vi "Set Goal A.vi"(11 "GIC Input":T1={"     Use ?\nOff       On"=[FALSE, TRUE, FALSE, TRUE], "Mode:"=FALSE, "Extra Port"="", "Hokuyo Port"="COM7", "Tx Prop  Port"="COM6", "Compass Port"="", "GPS Port"="", "Num of WPs"=0, "WP Lats and Longs"={"WP Lats"=[], "WP Longs"=[]}, "Obst Lats and Longs"={"Obst Lats"=[], "Obst Longs"=[]}, "Parameters"=[], "GPS Data"=[], "Compass"=0.0, "LMS Vector"=[], "Vision Vector"=[], "Direction Cmd"=0.0, "Speed Cmd"=0.0, "WP Vector"=[], "WP Number"=0, "Extra"=0, "SW Map"=[], "Path Cluster"={"Path x node"=[], "Path y node"=[]}, "Sim Course"=[]} {"Obst Lats and Longs"."Obst Longs" format="%#_8g"; "Obst Lats and Longs"."Obst Lats" format="%#_8g"}) -> (3 "GIC Output":T1={"     Use ?\nOff       On"=[FALSE, TRUE, FALSE, TRUE], "Mode:"=FALSE, "Extra Port"="", "Hokuyo Port"="COM7", "Tx Prop  Port"="COM6", "Compass Port"="", "GPS Port"="", "Num of WPs"=0, "WP Lats and Longs"={"WP Lats"=[], "WP Longs"=[]}, "Obst Lats and Longs"={"Obst Lats"=[], "Obst Longs"=[]}, "Parameters"=[], "GPS Data"=[], "Compass"=0.0, "LMS Vector"=[], "Vision Vector"=[], "Direction Cmd"=0.0, "Speed Cmd"=0.0, "WP Vector"=[], "WP Number"=0, "Extra"=0, "SW Map"=[], "Path Cluster"={"Path x node"=[], "Path y node"=[]}, "Sim Course"=[]} {"Obst Lats and Longs"."Obst Longs" format="%#_8g"; "Obst Lats and Longs"."Obst Lats" format="%#_8g"})   [LabVIEW 2014]
panel:
  out "tp":dbl
  out "wp vector":dbl[](array[numeric])
  out "test":dbl
  out "goal y":dbl
  in  "WP Vector":dbl[](array[numeric])=[-30.0, 100.0]
  out "goal x":dbl
  out "Test Output SWMap":dbl[][](array[numeric])
  in  "WayPoint:":dbl=100.0
  in  "Distance:":dbl=50.0
  in  "Slant:":dbl
  in  "Gap:":dbl=50.0
  in  "Ahead:":dbl
  # "Set Goal A"
  # "Input:"
  # "Output:"
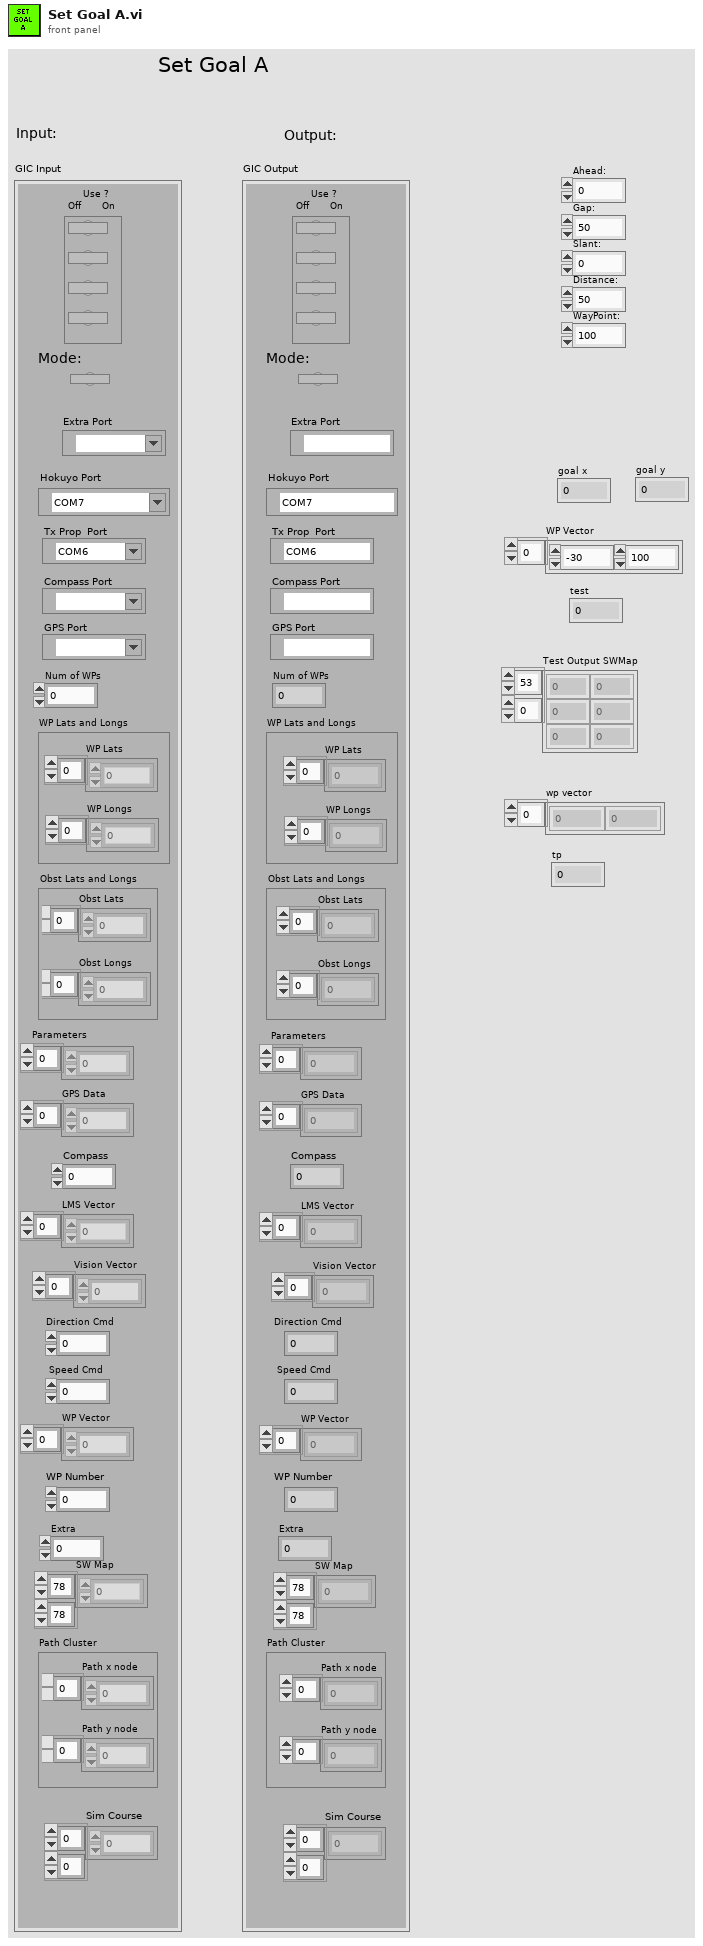
[diagram p1: front panel]
types:
  T1 = cluster{"     Use ?\nOff       On":bool[], "Mode:":bool, "Extra Port":refnum<visa-resource-name>, "Hokuyo Port":refnum<visa-resource-name>, "Tx Prop  Port":refnum<visa-resource-name>, "Compass Port":refnum<visa-resource-name>, "GPS Port":refnum<visa-resource-name>, "Num of WPs":i16, "WP Lats and Longs":cluster{"WP Lats":dbl[], "WP Longs":dbl[]}, "Obst Lats and Longs":cluster{"Obst Lats":dbl[], "Obst Longs":dbl[]}, "Parameters":dbl[], "GPS Data":dbl[], "Compass":dbl, "LMS Vector":dbl[], "Vision Vector":dbl[], "Direction Cmd":dbl, "Speed Cmd":dbl, "WP Vector":dbl[], "WP Number":i32, "Extra":i16, "SW Map":i32[][], "Path Cluster":cluster{"Path x node":dbl[], "Path y node":dbl[]}, "Sim Course":i8[][]}
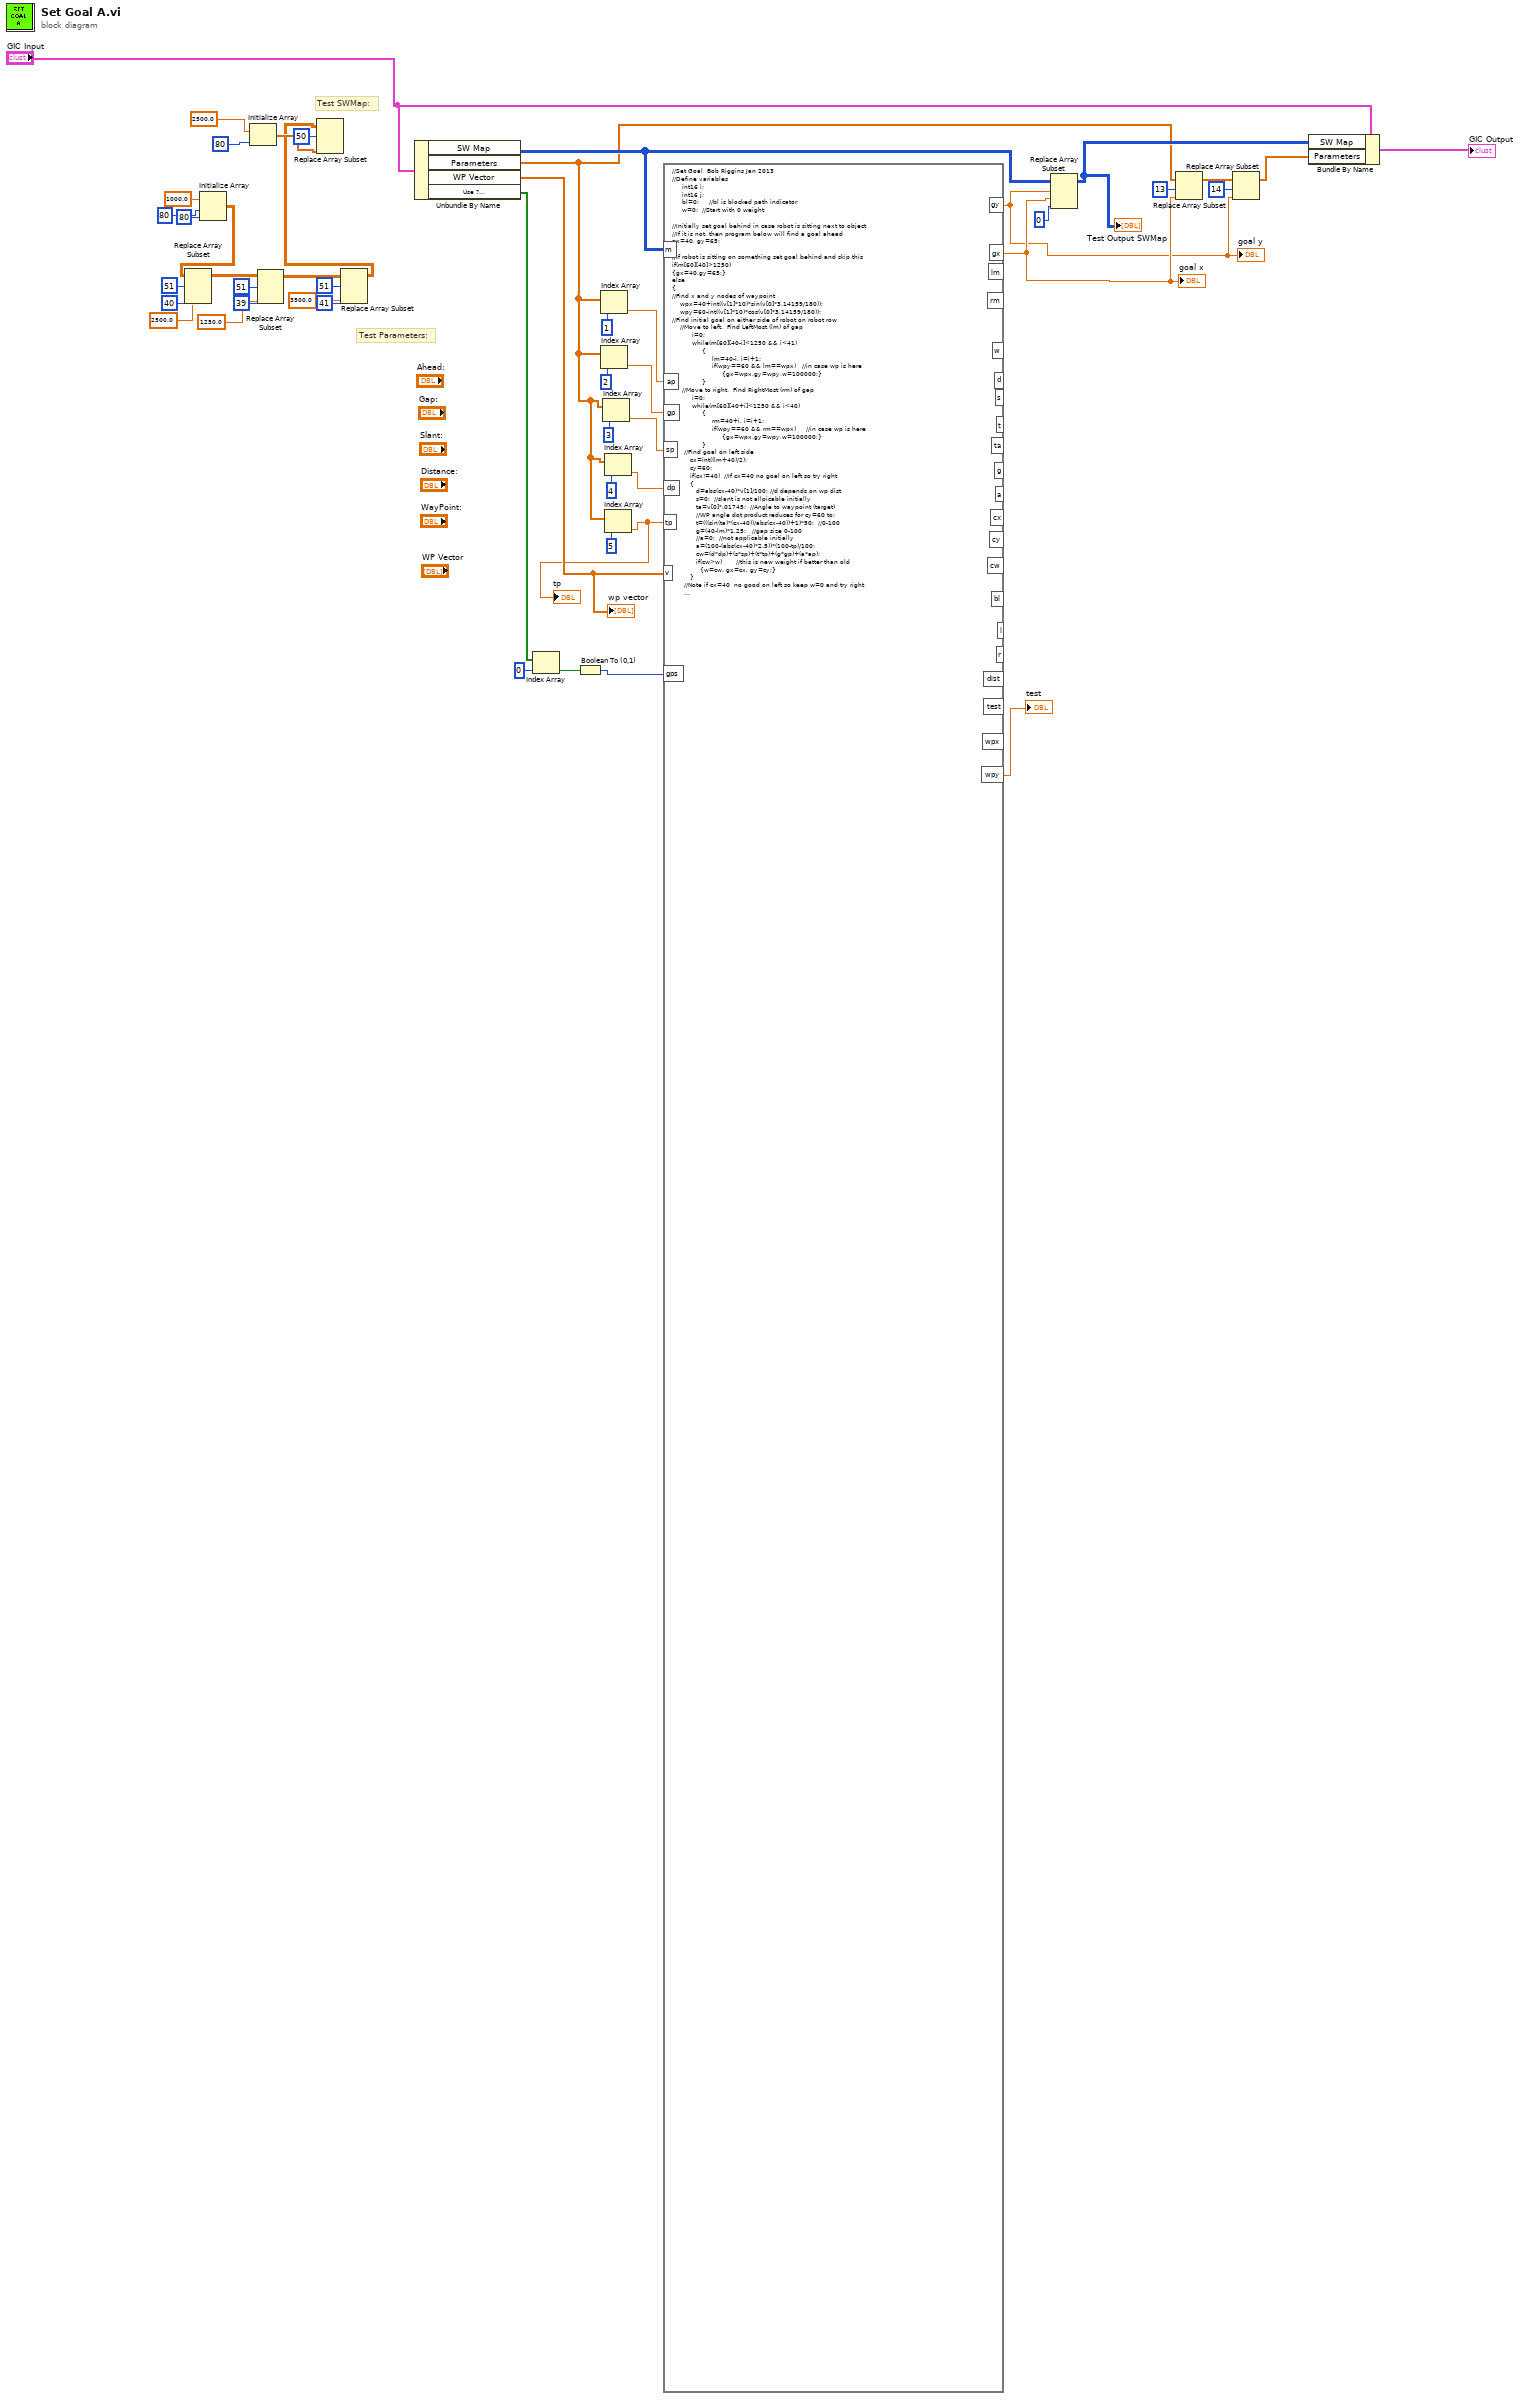
[diagram p0: block diagram]
diagram:
  # "Test Parameters:"
  # "Test SWMap:"
  n1 = Initialize Array(1000.0 ("element"), 80 ("dimension size"), 80 ("dimension size")) -> (w29:dbl[][])
  n2 = Replace Array Subset(array=w29, new element=2500.0 ("new element/subarray"), index (row)=51, index (col)=40 ("disabled index (col)")) -> (w42:dbl[][])
  n3 = Initialize Array(2500.0 ("element"), 80 ("dimension size")) -> (w31:dbl[])
  n4 = Replace Array Subset(array=w42, new element=1250.0 ("new element/subarray"), index (row)=51, index (col)=39 ("disabled index (col)")) -> (w38:dbl[][])
  n5 = Replace Array Subset(array=w38, new element=3500.0 ("new element/subarray"), index (row)=51, index (col)=41 ("disabled index (col)")) -> (w28:dbl[][])
  n6 = Replace Array Subset(array=w28, new element=w31, index (row)=50) -> ()  [unwired: 1 in, 1 out]
  n7 = Unbundle By Name("GIC Input") -> ("SW Map"=w25:i32[][], "Parameters"=w15:dbl[], "WP Vector"=w8:dbl[], "Use ?\nOff       On"=w6:bool[])
  "wp vector" <- w8
  n8 = Index Array(array=w6, index=0) -> (element=w4:bool)
  n9 = Boolean To (0,1)(Boolean=w4) -> (0, 1=w3:i16)
  n10 = Index Array(array=w15, index=1) -> (element=w24:dbl)
  n11 = Index Array(array=w15, index=2) -> (element=w21:dbl)
  n12 = Index Array(array=w15, index=3) -> (element=w19:dbl)
  n13 = Index Array(array=w15, index=4) -> (element=w17:dbl)
  n14 = Index Array(array=w15, index=5) -> (element=w7:dbl)
  "tp" <- w7
  n15 = formula code="//Set Goal  Bob Riggins Jan 2013\n//Define variables\n     int16 i;\n     int16 j;\n     bl=0;     //bl is blocked path indicator\n     w=0;  //Start with 0 weight\n\n//Initially set goal behind in case robot is sitting next to object\n//If it is not, then program below will find a goal ahead\ngx=40, gy=65;\n\n//If robot is sitting on something set goal behind and skip this\nif(m[60][40]>1250)\n{gx=40,gy=65;}\nelse\n{\n//Find x and y nodes of waypoint\n    wpx=40+int((v[1]*10)*sin(v[0]*3.14159/180));\n    wpy=60-int((v[1]*10)*cos(v[0]*3.14159/180));\n//Find initial goal on either side of robot on robot row\n    //Move to left.  Find LeftMost (lm) of gap\n          i=0;\n          while(m[60][40-i]<1250 && i<41)\n               {\n                    lm=40-i, i=i+1;\n                    if(wpy==60 && lm==wpx)   //in case wp is here\n                         {gx=wpx,gy=wpy,w=100000;}\n               }\n     //Move to right.  Find RightMost (rm) of gap\n          i=0;\n          while(m[60][40+i]<1250 && i<40)\n               {\n                    rm=40+i, i=i+1;\n                    if(wpy==60 && rm==wpx)     //in case wp is here\n                         {gx=wpx,gy=wpy,w=100000;}\n               }\n      //Find goal on left side\n         cx=int((lm+40)/2);\n         cy=60;\n         if(cx!=40)  //If cx=40 no goal on left so try right\n         {\n            d=abs(cx-40)*v[1]/100; //d depends on wp dist\n            s=0;  //slant is not allpicable initially\n            ta=v[0]*.01745;  //Angle to waypoint (target)\n            //WP angle dot product reduces for cy=60 to:\n            t=(((sin(ta)*(cx-40))/abs(cx-40))+1)*50;  //0-100\n            g=(40-lm)*1.25;   //gap size 0-100\n            //a=0;  //not applicable initially\n            a=(100-(abs(cx-40)*2.5))*(100-tp)/100;\n            cw=(d*dp)+(s*sp)+(t*tp)+(g*gp)+(a*ap);\n            if(cw>w)       //this is new weight if better than old\n              {w=cw, gx=cx, gy=cy;} \n         }\n      //Note if cx=40  no good on left so keep w=0 and try right\n      //Find candidate goal on right side\n         cx=int((40+rm)/2);  \n         cy=60;\n         if(cx!=40)  //If cx=40 no goal on right so dont even try\n         {\n              d=abs(cx-40)*v[1]/100;  \n              s=0;  //slant is not allpicable initially\n              ta=v[0]*.01745;  //Angle to waypoint (target)\n              //WP angle dot product reduces for gy=60 to:\n              t=(((sin(ta)*(cx-40))/abs(cx-40))+1)*50;  //0-100\n              g=(rm-40)*1.25;   //gap size 0-100\n              //a=0;  //not applicable initially\n              a=(100-(abs(cx-40)*2.5))*(100-tp)/100;\n              cw=(d*dp)+(s*sp)+(t*tp)+(g*gp)+(a*ap);\n              if(cw>w)       //change goal if the right is better\n                   {w=cw, gx=cx, gy=cy;} \n         }    \n\n//Main Loop, move up row by row checking candidates\n//Candidate goals are midpoints and both edges of all gaps\n     cy=60;\n     while(cy>0&&bl==0)\n     {\n      //start scout one row up and 1 to left unless on edge\n           if(lm==0)\n                {cx=0;}\n           else\n                {cx=lm-1;}\n           cy=cy-1; \n      //move scout to right until on clear node\n           while(m[int(cy)][int(cx)]>1249 && cx<80)\n                {cx=cx+1;}\n           if(cx==80||cx>rm+1)\n            {bl=1;  }   //means this row is blocked--can quit looking  \n      //move scout to left until on occupied node--make new lm\n           while(m[int(cy)][int(cx)]<1250 && cx>0 && bl==0)\n                {\n                    cx=cx-1;\n                    if(cy==wpy && cx==wpx)     //in case wp is here\n                         {gx=wpx,gy=wpy,w=100000;}\n                }\n           cx=cx+1;\n           lm=cx;       //new lm\n           l=lm;              //l is left of first gap on row\n      //Find all gaps on row by finding l and r of each\n      //l of first gap already found above (l=lm)\n           i=lm;  //start scout i at lm\n           while(i<80 && bl==0)   //move across row to find all gaps  \n                {\n                     while(m[int(cy)][i]<1250 && i<80)\n                          {\n                               i=i+1;\n                               if(cy==wpy && i==wpx)     //in case wp is here\n                                    {gx=wpx,gy=wpy,w=100000;}\n                          }\n                     if(i==80)\n                          {rm=79, r=rm;}\n                     else\n                          {r=i-1;}   //we now have l and r of this gap\n\n                     //Next search for best goal so far in this gap\n                     //Set goal only in middlepoint unless on edge and\n                     //unless use gps\n\n                     if(cy==0 && gps==1)\n                     {\n                          for(cx=l;cx<=r;cx=cx+1)\n                          {\n                               dist=((cx-40)**2+(cy-60)**2)**.5;\n                               d=dist*v[1]/100; \n                               ta=v[0]*.01745;  //Angle to waypoint (target)\n                               t=((((cx-40)*sin(ta)+(60-cy)*cos(ta))/dist)+1)*50;\n                               g=(r-l)*1.25;   //gap size 0-100\n                               //a=0;  //not applicable initially \n                               a=(100-(abs(cx-40)*2.5))*(100-tp)/100;\n                               cw=(d*dp)+(s*sp)+(t*tp)+(g*gp)+(a*ap);\n                               if(cw>w)       //change goal if it beats all before\n                                    {w=cw, gx=cx, gy=cy;}\n                          } \n                     }\n                     else\n                     {\n                          cx=int((l+r)/2);\n                          dist=((cx-40)**2+(cy-60)**2)**.5;\n                          d=dist*v[1]/100; \n                          ta=v[0]*.01745;  //Angle to waypoint (target)\n                          t=((((cx-40)*sin(ta)+(60-cy)*cos(ta))/dist)+1)*50;\n                          //g=(r-l)*1.25;   //gap size 0-100\n                          if(l>0 && r<79)\n                          {\n                               if(r-l<=60)\n                                    {g=100-(abs(r-l-30)*3.33);}\n                               else\n                                    {g=0;}\n                          }\n                          else\n                               {g=0;}\n                          //a=0;  //not applicable initially \n                          a=(100-(abs(cx-40)*2.5))*(100-tp)/100;\n                          cw=(d*dp)+(s*sp)+(t*tp)+(g*gp)+(a*ap);\n                          if(cw>w)       //change goal if it beats all before\n                               {w=cw, gx=cx, gy=cy;}\n                     } \n                     cx=r;\n                     //Move scout to right to find L of next gap     \n                          while(m[int(cy)][i]>1249 && i<80)\n                               {i=i+1; }\n                     //Dont check any more gaps on row if i>rm+1\n                        if(i>rm+1)\n                             {i=80;}\n                        if(i<80)\n                             {l=i;}\n\n                }    //end of while checking for all gaps on a row\n                rm=r;   //right max is last right on row\n   }    //end of main loop moving to top of map\n}  //End of big if to see if robot is sitting on something"("m"=w25, "ap"=w24, "gp"=w21, "sp"=w19, "dp"=w17, "tp"=w7, "v"=w8, "gps"=w3) -> ("gx"=w13:dbl, "gy"=w10:dbl, "wpy"=→"test":dbl)  [unwired: 18 out]
  "goal x" <- w13
  "goal y" <- w10
  n16 = Replace Array Subset(array=w25, new element=0 ("new element/subarray"), index (row)=w10, index (col)=w13) -> (w27:i32[][])
  "Test Output SWMap" <- w27
  n17 = Replace Array Subset(array=w15, new element=w13, index=13) -> (w12:dbl[])
  n18 = Replace Array Subset(array=w12, new element=w10, index=14) -> (w9:dbl[])
  n19 = Bundle By Name(cluster="GIC Input", "SW Map"=w27, "Parameters"=w9) -> (→"GIC Output":T1)
